vi "BuildProcess.vi"() -> ()   [LabVIEW 2016]
uses:
  BuildItem.ctl
  <vilib>/Utility/error.llb/Error Cluster From Error Code.vi
  <vilib>/ErrorRing/Error Ring.xnode
  <vilib>/addons/_JKI.lib/Serialization/JSON/JKI JSON Serialization.lvlib
panel:
  in  "Workspace path":path=path "C:/temp/Workspace"
  in  "Clean Cache?":bool
  in  "CleanCodebase":bool=TRUE
  in  "CheckSystemComponents":bool
  in  "FetchCodebase?":bool
  out "String":string
  out "error out":errorcluster
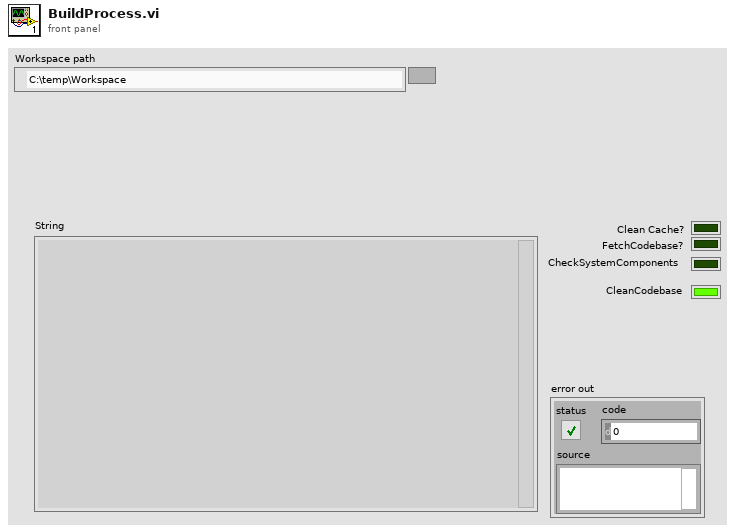
[diagram p1: front panel]
types:
  T1 = typedef "BuildItem.ctl" = cluster{"Project":path, "BuildSpecification":path, "Destination":path}
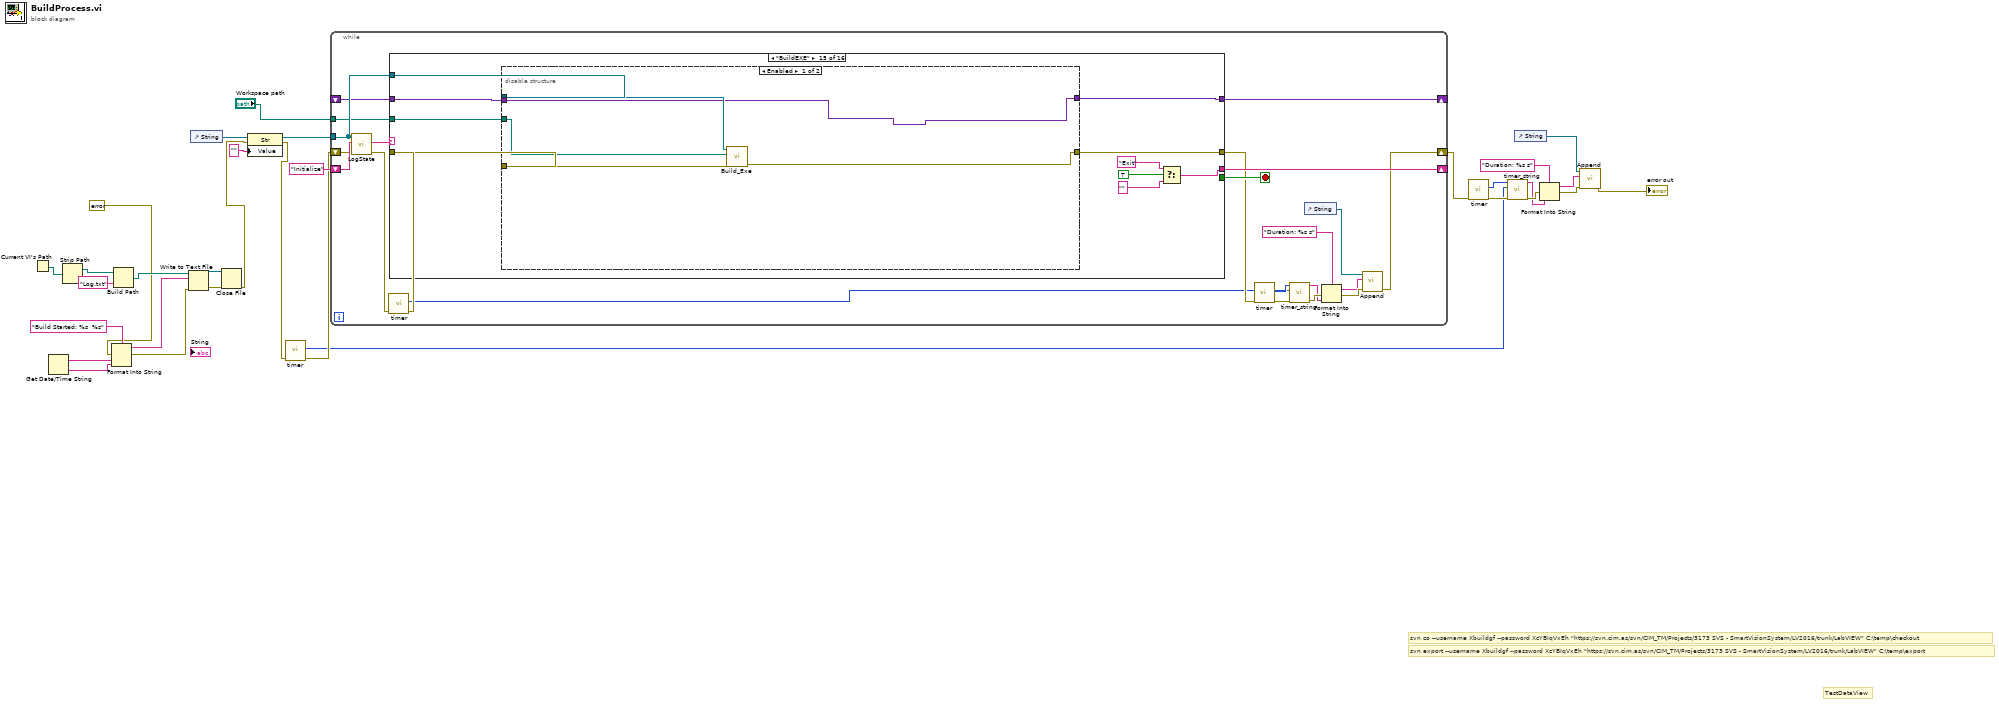
[diagram p0: block diagram]
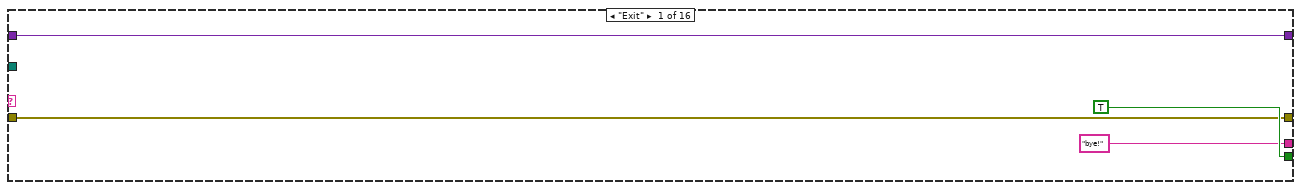
[diagram p2: hidden frame]
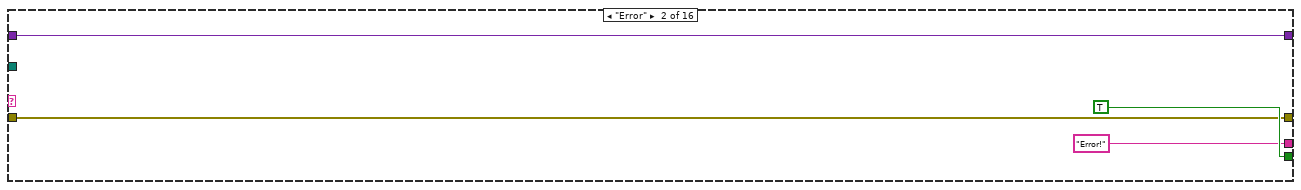
[diagram p3: hidden frame]
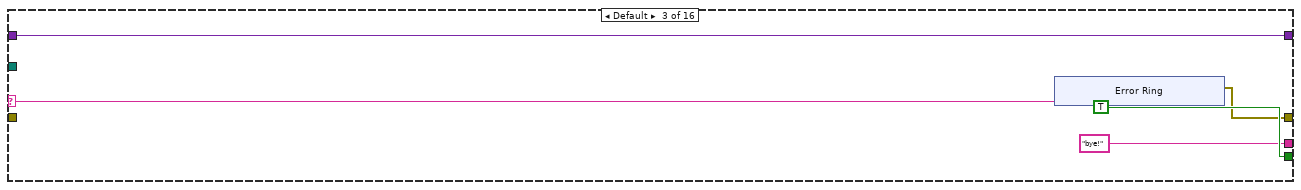
[diagram p4: hidden frame]
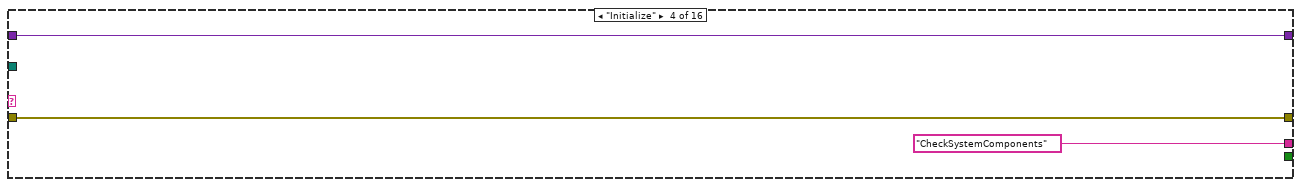
[diagram p5: hidden frame]
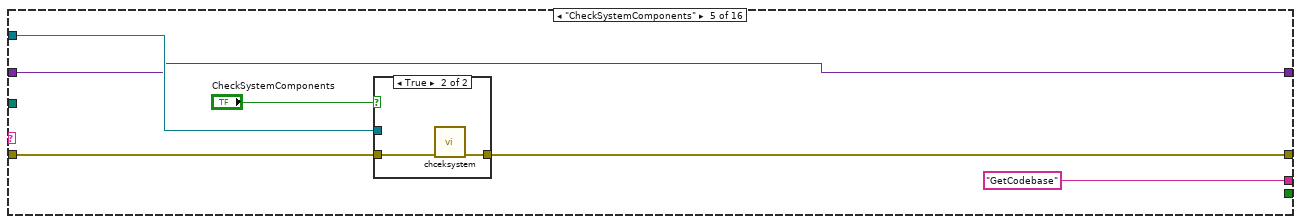
[diagram p6: hidden frame]
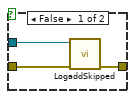
[diagram p7: hidden frame]
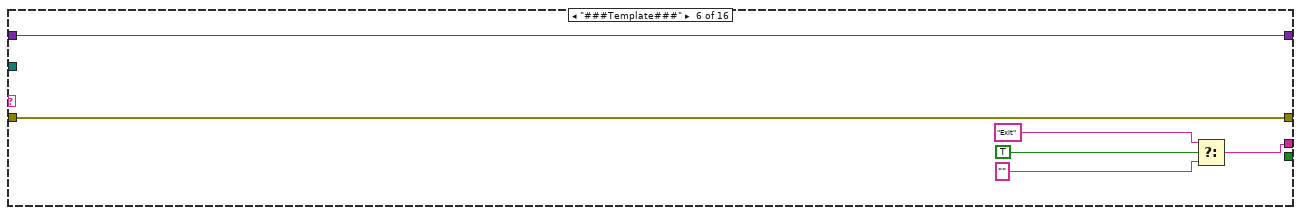
[diagram p8: hidden frame]
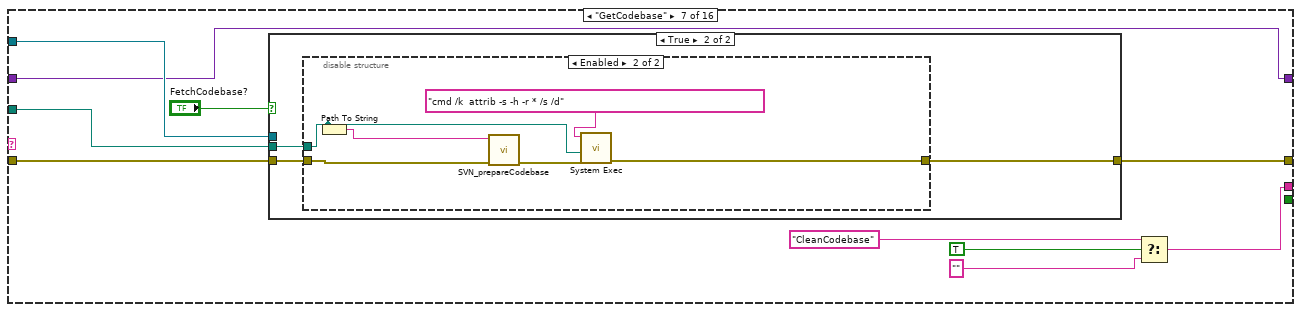
[diagram p9: hidden frame]
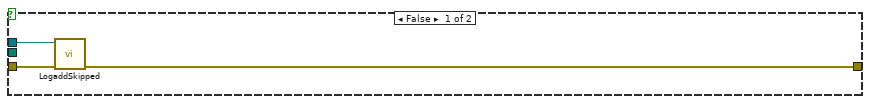
[diagram p10: hidden frame]
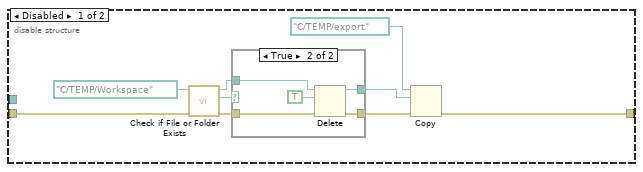
[diagram p11: hidden frame]
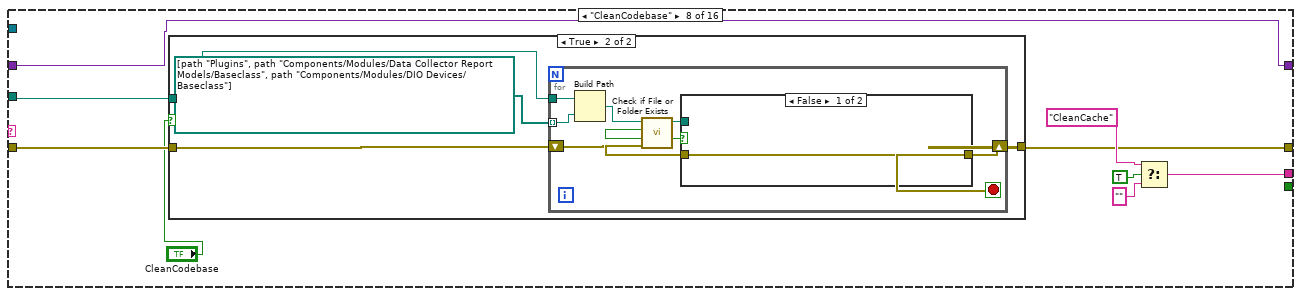
[diagram p13: hidden frame]
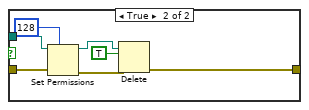
[diagram p15: hidden frame]
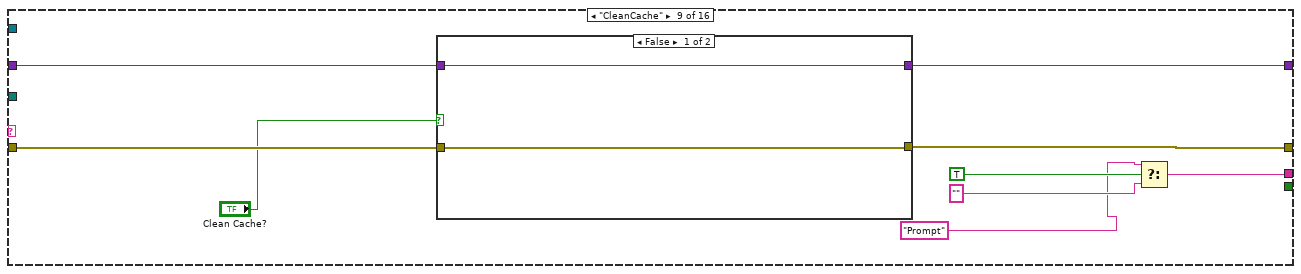
[diagram p16: hidden frame]
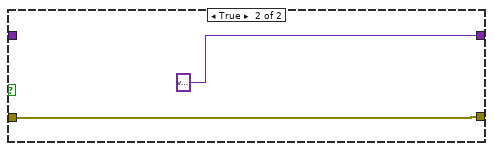
[diagram p17: hidden frame]
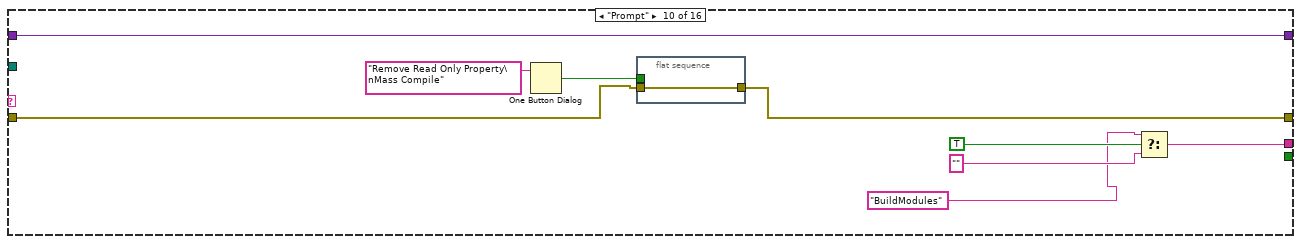
[diagram p18: hidden frame]
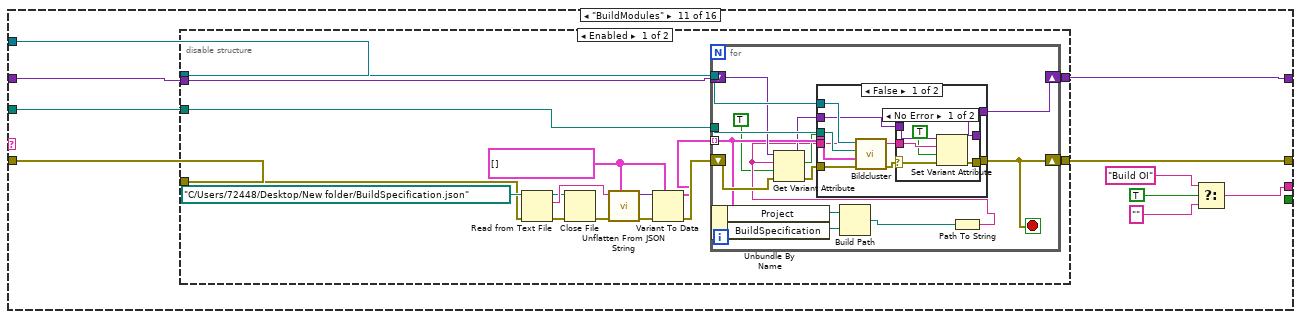
[diagram p19: hidden frame]
diagram:
  # "TestDataView"
  # "svn co --username Xbuildgf --password XcYBIqVxEh \"https://svn.cim.as/svn/CIM_TM/Projects/3173 SVS - SmartVisionSystem/LV2016/trunk/LabVIEW\" C:\\temp\\checkout"
  # "svn export --username Xbuildgf --password XcYBIqVxEh \"https://svn.cim.as/svn/CIM_TM/Projects/3173 SVS - SmartVisionSystem/LV2016/trunk/LabVIEW\" C:\\temp\\export"
  n1 = Current VI's Path() -> (path=w13:path)
  n2 = Get Date/Time String() -> (date string=w4:string, time string=w3:string)  [unwired: 3 in]
  n3 = Strip Path(path=w13) -> (stripped path=w12:path)  [unwired: 1 out]
  n4 = Format Into String(format string="Build Started: %s  %s", error in=errorcluster {"status"=FALSE, "code"=0, "source"=""} ("error out"), w4, w3) -> (resulting string=w5:string, error out=w1:errorcluster)  [unwired: 1 in]
  n5 = Build Path(base path=w12, name or relative path="Log.txt") -> (appended path=w11:path)
  n6 = Write to Text File(file (use dialog)=w11, text=w5, error in=w1) -> (refnum out=w10:refnum<file>, error out=w9:errorcluster)  [unwired: 1 in, 1 out]
  n7 = control-ref of="String"() -> (w30:refnum<vi>)
  n8 = Close File(refnum=w10, error in=w9) -> (error out=w7:errorcluster)  [unwired: 1 out]
  n9 = property class="Str"(reference=w30, error in=w7, "Value"="") -> (reference out=w29:refnum<vi>, error out=w26:errorcluster)
  n10 = call "timer.vi"("error in (no error)"=w26) -> ("error out"=w25:errorcluster, "millisecond timer value"=w18:u32)  [unwired: 9 in]
  n11 = while {
    shift-right: [w52] -> _
    shift-left: "Initialize" -> [w51]
    shift-right: [w36] -> w23
    shift-left: w25 -> [w49]
    tunnel: w29 -> [w48]
    shift-right: [w46] -> _
    shift-left: _ -> [w47]
    tunnel: "Workspace path" -> [w45]
    stop <- w53 stop-if-true
    n12 = call "LogState.vi"("error in (no error)"=w49, "State In"=w51, "String in"=w48) -> ("error out"=w44:errorcluster, "State Out"=w50:string)  [unwired: 7 in]
    n13 = call "timer.vi"("error in (no error)"=w44) -> ("error out"=w43:errorcluster, "millisecond timer value"=w39:u32)  [unwired: 9 in]
    n14 = case shown="\"BuildEXE\"" w50 {
      selector: w50 -> [_ _ w64 _ _ _ _ _ _ _ _ _ _ _ _ _]
      tunnel: [TRUE TRUE TRUE _ _ _ _ _ _ _ _ _ _ _ _ _] -> w53
      tunnel: ["bye!" "Error!" "bye!" "CheckSystemComponents" "GetCodebase" w92 w102 w140 w170 w183 w193 w259 w283 w307 w327 w344] -> w52
      tunnel: [w55 w59 w63 w76 w81 w90 w99 w133 w166 w176 w190 w255 w279 w303 w324 w341] -> w42
      tunnel: w43 -> [w55 w59 _ w76 w80 w90 w98 w137 w167 w177 w188 w254 w278 w302 w322 w339]
      tunnel: w48 -> [_ _ _ _ w78 _ w96 _ _ _ w189 _ _ _ w323 w340]
      tunnel: w47 -> [w54 w58 w62 w74 w77 w88 w95 w134 w162 w179 w187 w249 w274 w298 w321 w338]
      tunnel: [w54 w58 w62 w74 w77 w88 w95 w134 w163 w179 w186 w248 w273 w297 w320 w337] -> w46
      tunnel: w45 -> [_ _ _ _ _ _ w94 w132 _ _ w185 w256 w280 w304 w319 w336]
      frame "Exit" {
      }
      frame "Error" {
      }
      frame Default {
        n15 = xnode "Error Ring"("parameter 0"=w64) -> ("error out"=w63:errorcluster)
      }
      frame "Initialize" {
      }
      frame "CheckSystemComponents" {
        n16 = case shown="True" "CheckSystemComponents" {
          tunnel: [w84 w87] -> w81
          tunnel: w80 -> [w85 w86]
          tunnel: w78 -> [w83 _]
          frame False {
            n17 = call "LogaddSkipped.vi"("error in (no error)"=w85, "String in"=w83) -> ("error out"=w84:errorcluster)  [unwired: 9 in]
          }
          frame True {
            n18 = call "chceksystem.vi"("error in (no error)"=w86) -> ("Error out"=w87:errorcluster)  [unwired: 8 in, 2 out]
          }
        }
      }
      frame "###Template###" {
        n19 = Select(t="Exit", s=TRUE, f="") -> (s? t:f=w92:string)
      }
      frame "GetCodebase" {
        n20 = case shown="True" "FetchCodebase?" {
          tunnel: [w104 w109] -> w99
          tunnel: w98 -> [w106 w108]
          tunnel: w96 -> [w105 _]
          tunnel: w94 -> [_ w107]
          frame False {
            n21 = call "LogaddSkipped.vi"("error in (no error)"=w106, "String in"=w105) -> ("error out"=w104:errorcluster)  [unwired: 9 in]
          }
          frame True {
            n22 = disable-structure shown="Enabled" {
              disable-tunnel: [w118 w128] -> w109
              disable-tunnel: w108 -> [w117 w131]
              disable-tunnel: w107 -> [_ w126]
              frame Disabled {
                n23 = call <vilib>:"Check if File or Folder Exists.vi"("error in (no error)"=w117, "path"=path "C:/TEMP/Workspace" ("target path (use dialog)")) -> ("error out"=w111:errorcluster, "file or folder exists?"=w110:bool, "dup path"=w112:path)  [unwired: 7 in]
                n24 = case shown="True" w110 {
                  tunnel: [w119 w125] -> w115
                  tunnel: [w120 w123] -> w114
                  tunnel: w112 -> [w120 w122]
                  tunnel: w111 -> [w119 w121]
                  frame False {
                  }
                  frame True {
                    n25 = Delete(path (use dialog)=w122, entire hierarchy (F)=TRUE, error in=w121) -> (deleted path=w123:path, error out=w125:errorcluster)  [unwired: 2 in, 1 out]
                  }
                }
                n26 = Copy(8:w115, 10:w114, 11:path "C:/TEMP/export" ("source path")) -> (0:w118:errorcluster)  [unwired: 2 in, 2 out]
              }
              frame Enabled {
                n27 = Path To String(path=w126) -> (string=w130:string)
                n28 = call "SVN_prepareCodebase.vi"("error in (no error)"=w131, "Path"=w130) -> ("error out"=w129:errorcluster)  [unwired: 6 in, 3 out]
                n29 = call <vilib>:"System Exec.vi"("error in (no error)"=w129, "working directory"=w126, "command line"="cmd /k  attrib -s -h -r * /s /d") -> ("error out"=w128:errorcluster)  [unwired: 5 in, 3 out]
              }
            }
          }
        }
        n30 = Select(t="CleanCodebase", s=TRUE, f="") -> (s? t:f=w102:string)
      }
      frame "CleanCodebase" {
        n31 = case shown="True" "CleanCodebase" {
          tunnel: w137 -> [w141 w145]
          tunnel: [w141 w144] -> w133
          tunnel: w132 -> [_ w142]
          frame False {
          }
          frame True {
            n32 = for {
              shift-right: [w149] -> w144
              shift-left: w145 -> [w150]
              tunnel: path[] [path "Plugins", path "Components/Modules/Data Collector Report Models/Baseclass", path "Components/Modules/DIO Devices/Baseclass"] -> [w147] mode=indexing
              tunnel: w142 -> [w148]
              stop <- w149 stop-if-true
              n33 = Build Path(base path=w148, name or relative path=w147) -> (appended path=w146:path)
              n34 = call <vilib>:"Check if File or Folder Exists.vi"("error in (no error)"=w150, "path"=w146) -> ("error out"=w152:errorcluster, "file or folder exists?"=w151:bool, "dup path"=w153:path)  [unwired: 7 in]
              n35 = case shown="False" w151 {
                tunnel: [w154 w161] -> w149
                tunnel: w153 -> [_ w158]
                tunnel: w152 -> [w154 w159]
                frame False {
                }
                frame True {
                  n36 = Set Permissions(7:i16 128 ("permissions"), 8:w159, 11:w158) -> (0:w156:errorcluster, 3:w155:path)  [unwired: 2 in]
                  n37 = Delete(path (use dialog)=w155, entire hierarchy (F)=TRUE, error in=w156) -> (error out=w161:errorcluster)  [unwired: 2 in, 2 out]
                }
              }
            }
          }
        }
        n38 = Select(t="CleanCache", s=TRUE, f="") -> (s? t:f=w140:string)
      }
      frame "CleanCache" {
        n39 = case shown="False" "Clean Cache?" {
          tunnel: w167 -> [w172 w174]
          tunnel: [w172 w174] -> w166
          tunnel: [w171 variant] -> w163
          tunnel: w162 -> [w171 _]
          frame False {
          }
          frame True {
          }
        }
        n40 = Select(t="Prompt", s=TRUE, f="") -> (s? t:f=w170:string)
      }
      frame "Prompt" {
        n41 = One Button Dialog(message="Remove Read Only Property\nMass Compile") -> (true=w178:bool)  [unwired: 1 in]
        n42 = flat-sequence {
          tunnel: w178 -> [_]
          tunnel: w177 -> [w184]
          tunnel: [w184] -> w176
          frame #0 {
          }
        }
        n43 = Select(t="BuildModules", s=TRUE, f="") -> (s? t:f=w183:string)
      }
      frame "BuildModules" {
        n44 = disable-structure shown="Enabled" {
          disable-tunnel: [w210 w246] -> w190
          disable-tunnel: w189 -> [w209 _]
          disable-tunnel: w188 -> [w200 w246]
          disable-tunnel: w187 -> [w197 w245]
          disable-tunnel: [w196 w245] -> w186
          disable-tunnel: w185 -> [w195 _]
          frame Enabled {
            w207 = T1[] []
            n45 = Read from Text File(file (use dialog)=path "C:/Users/72448/Desktop/New folder/BuildSpecification.json", error in=w200) -> (refnum out=w201:refnum<file>, text=w204:string, error out=w202:errorcluster)  [unwired: 2 in, 1 out]
            n46 = Close File(refnum=w201, error in=w202) -> (error out=w203:errorcluster)  [unwired: 1 out]
            n47 = call <vilib>:"Unflatten From JSON String.vi"("Type and Defaults"=w207, "error in (no error)"=w203, "JSON String"=w204) -> ("error out"=w208:errorcluster, "Variant"=w206:variant)  [unwired: 7 in]
            n48 = Variant To Data(error in=w208, type=w207, Variant=w206) -> (data=w198:T1[], error out=w199:errorcluster)
            n49 = for {
              tunnel: w195 -> [w225]
              tunnel: w209 -> [w224]
              shift-right: [w211] -> w210
              shift-left: w199 -> [w223]
              tunnel: w198 -> [w221] mode=indexing
              shift-right: [w215] -> w196
              shift-left: w197 -> [w222]
              stop <- w211 stop-if-true
              n50 = Unbundle By Name(w221) -> ("Project"=w220:path, "BuildSpecification"=w219:path)
              n51 = Build Path(base path=w220, name or relative path=w219) -> (appended path=w218:path)
              n52 = Path To String(path=w218) -> (string=w213:string)
              n53 = Get Variant Attribute(Variant=w222, name=w213, default value (empty Variant)=TRUE, error in=w223) -> (duplicate Variant=w214:variant, found=w216:bool, error out=w217:errorcluster)  [unwired: 1 out]
              n54 = case shown="False" w216 {
                tunnel: [w229 w244] -> w211
                tunnel: w225 -> [w234 _]
                tunnel: w224 -> [w233 _]
                tunnel: w221 -> [w232 _]
                tunnel: w217 -> [w231 w244]
                tunnel: [w227 w243] -> w215
                tunnel: w214 -> [w228 w243]
                tunnel: w213 -> [w226 _]
                frame False {
                  n55 = call "Bildcluster.vi"("error in (no error)"=w231, "BuildItem"=w232, "path"=w234, "String in"=w233) -> ("error out"=w230:errorcluster)  [unwired: 7 in]
                  n56 = case shown="No Error" w230 {
                    selector: w230 -> [w237 w241]
                    tunnel: [w236 w241] -> w229
                    tunnel: w228 -> [w240 w242]
                    tunnel: [w239 w242] -> w227
                    tunnel: w226 -> [w238 _]
                    frame No Error {
                      n57 = Set Variant Attribute(Variant=w240, name=w238, value=TRUE, error in=w237) -> (Variant out=w239:variant, error out=w236:errorcluster)  [unwired: 1 out]
                    }
                    frame Error {
                    }
                  }
                }
                frame True {
                }
              }
            }
          }
          frame Disabled {
          }
        }
        n58 = Select(t="Build OI", s=TRUE, f="") -> (s? t:f=w193:string)
      }
      frame "Build OI" {
        w252 = "Components\\OIs\\Build all OI projects.vi" ("name or relative path")
        n59 = Get Variant Attribute(Variant=w249, name=w252, default value (empty Variant)=TRUE, error in=w254) -> (duplicate Variant=w251:variant, found=w247:bool, error out=w250:errorcluster)  [unwired: 1 out]
        n60 = case shown="False" w247 {
          selector: w247 -> [w265 _]
          tunnel: w256 -> [w268 _]
          tunnel: [w262 w269] -> w255
          tunnel: w252 -> [w264 _]
          tunnel: w251 -> [w266 w270]
          tunnel: w250 -> [w263 w269]
          tunnel: [w261 w270] -> w248
          frame False {
            n61 = call "run_BuildAll.vi"("error in (no error)"=w263, "name or relative path"=w264, "Workspace path"=w268) -> ("error out"=w267:errorcluster)  [unwired: 8 in]
            n62 = Set Variant Attribute(Variant=w266, name=w264, value=w265, error in=w267) -> (Variant out=w261:variant, error out=w262:errorcluster)  [unwired: 1 out]
          }
          frame True {
          }
        }
        n63 = Select(t="BuildSequenceModules", s=TRUE, f="") -> (s? t:f=w259:string)
      }
      frame "BuildSequenceModules" {
        w272 = "Components\\Sequence Modules\\Build all Sequence Module projects.vi" ("name or relative path")
        n64 = Get Variant Attribute(Variant=w274, name=w272, default value (empty Variant)=TRUE, error in=w278) -> (duplicate Variant=w276:variant, found=w271:bool, error out=w275:errorcluster)  [unwired: 1 out]
        n65 = case shown="False" w271 {
          selector: w271 -> [w289 _]
          tunnel: w280 -> [w292 _]
          tunnel: [w286 w293] -> w279
          tunnel: w272 -> [w288 _]
          tunnel: w276 -> [w290 w294]
          tunnel: w275 -> [w287 w293]
          tunnel: [w285 w294] -> w273
          frame False {
            n66 = call "run_BuildAll.vi"("error in (no error)"=w287, "name or relative path"=w288, "Workspace path"=w292) -> ("error out"=w291:errorcluster)  [unwired: 8 in]
            n67 = Set Variant Attribute(Variant=w290, name=w288, value=w289, error in=w291) -> (Variant out=w285:variant, error out=w286:errorcluster)  [unwired: 1 out]
          }
          frame True {
          }
        }
        n68 = Select(t="BuildProcessModules", s=TRUE, f="") -> (s? t:f=w283:string)
      }
      frame "BuildProcessModules" {
        w296 = "Components\\Process Modules\\Build all Process Module projects.vi" ("name or relative path")
        n69 = Get Variant Attribute(Variant=w298, name=w296, default value (empty Variant)=TRUE, error in=w302) -> (duplicate Variant=w300:variant, found=w295:bool, error out=w299:errorcluster)  [unwired: 1 out]
        n70 = case shown="False" w295 {
          selector: w295 -> [w313 _]
          tunnel: w304 -> [w316 _]
          tunnel: [w310 w317] -> w303
          tunnel: w296 -> [w312 _]
          tunnel: w300 -> [w314 w318]
          tunnel: w299 -> [w311 w317]
          tunnel: [w309 w318] -> w297
          frame False {
            n71 = call "run_BuildAll.vi"("error in (no error)"=w311, "name or relative path"=w312, "Workspace path"=w316) -> ("error out"=w315:errorcluster)  [unwired: 8 in]
            n72 = Set Variant Attribute(Variant=w314, name=w312, value=w313, error in=w315) -> (Variant out=w309:variant, error out=w310:errorcluster)  [unwired: 1 out]
          }
          frame True {
          }
        }
        n73 = Select(t="MakeZipfile", s=TRUE, f="") -> (s? t:f=w307:string)
      }
      frame "BuildEXE" {
        n74 = disable-structure shown="Enabled" {
          disable-tunnel: [w329 w335] -> w324
          disable-tunnel: w323 -> [w333 _]
          disable-tunnel: w322 -> [w332 w335]
          disable-tunnel: w321 -> [w331 w334]
          disable-tunnel: [w331 w334] -> w320
          disable-tunnel: w319 -> [w330 _]
          frame Enabled {
            n75 = call "Build_Exe.vi"("error in (no error)"=w332, "Workspace path"=w330, "String in"=w333) -> ("error out"=w329:errorcluster)  [unwired: 8 in]
          }
          frame Disabled {
          }
        }
        n76 = Select(t="Exit", s=TRUE, f="") -> (s? t:f=w327:string)
      }
      frame "MakeZipfile" {
        n77 = disable-structure shown="Enabled" {
          disable-tunnel: [w346 w351] -> w341
          disable-tunnel: w340 -> [_ _]
          disable-tunnel: w339 -> [w347 w351]
          disable-tunnel: w338 -> [w349 w350]
          disable-tunnel: [w349 w350] -> w337
          disable-tunnel: w336 -> [w348 _]
          frame Enabled {
            n78 = call "ZipPlugins.vi"("error in (no error)"=w347, "Workspace path"=w348) -> ("error out"=w346:errorcluster)  [unwired: 9 in]
          }
          frame Disabled {
          }
        }
        n79 = Select(t="BuildEXE", s=TRUE, f="") -> (s? t:f=w344:string)
      }
    }
    n80 = call "timer.vi"("error in (no error)"=w42) -> ("error out"=w41:errorcluster, "millisecond timer value"=w40:u32)  [unwired: 9 in]
    n81 = call "timer_string.vi"("error in (no error)"=w41, "millisecond timer value"=w39, "millisecond timer value 2"=w40) -> ("error out"=w37:errorcluster, "String"=w35:string)  [unwired: 7 in]
    n82 = control-ref of="String"() -> (w32:refnum<vi>)
    n83 = Format Into String(format string="Duration: %s s", error in=w37, w35) -> (resulting string=w33:string, error out=w38:errorcluster)  [unwired: 1 in]
    n84 = call "Append.vi"("error in (no error)"=w38, "Msg in"=w33, "String in"=w32) -> ("error out"=w36:errorcluster)  [unwired: 7 in]
  }
  n85 = call "timer.vi"("error in (no error)"=w23) -> ("error out"=w19:errorcluster, "millisecond timer value"=w17:u32)  [unwired: 9 in]
  n86 = call "timer_string.vi"("error in (no error)"=w19, "millisecond timer value"=w18, "millisecond timer value 2"=w17) -> ("error out"=w20:errorcluster, "String"=w16:string)  [unwired: 7 in]
  n87 = control-ref of="String"() -> (w14:refnum<vi>)
  n88 = Format Into String(format string="Duration: %s s", error in=w20, w16) -> (resulting string=w15:string, error out=w21:errorcluster)  [unwired: 1 in]
  n89 = call "Append.vi"("error in (no error)"=w21, "Msg in"=w15, "String in"=w14) -> ("error out"=→"error out":errorcluster)  [unwired: 7 in]
